vi "Handle EStop.vi"(8 "error in (no error)":errorcluster, 10 "Temp. Input":dbl, 11 "Tag Name":string) -> (0 "error out":errorcluster, 2 "History Data":T1(array[cluster]))   [LabVIEW 2023]
uses:
  8fdf3798-820e-43b9-bbcf-a8150b0dfc24.vi
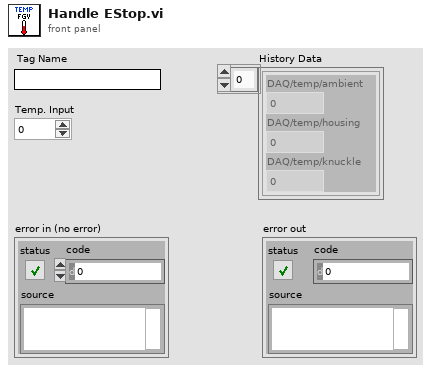
[diagram p1: front panel]
types:
  T1 = cluster{"DAQ/temp/ambient":dbl, "DAQ/temp/housing":dbl, "DAQ/temp/knuckle":dbl}[]
  T2 = cluster{"DAQ/temp/ambient":dbl, "DAQ/temp/housing":dbl, "DAQ/temp/knuckle":dbl}
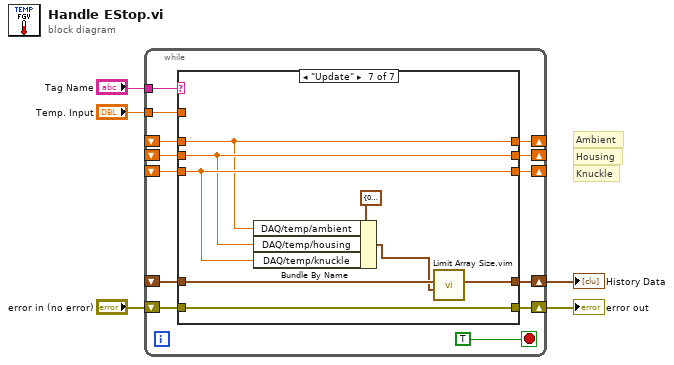
[diagram p0: block diagram]
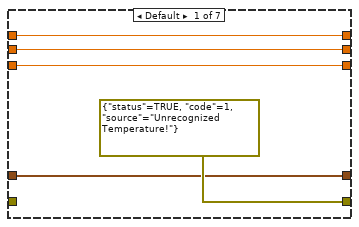
[diagram p2: hidden frame]
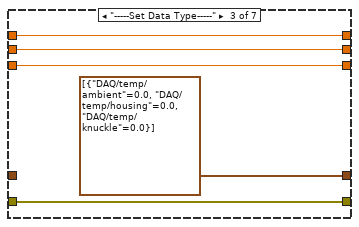
[diagram p4: hidden frame]
diagram:
  # "Knuckle"
  # "Housing"
  # "Ambient"
  n1 = while {
    tunnel: "Tag Name" -> [w14]
    shift-right: [w12] -> w2
    shift-left: _ -> [w13]
    shift-right: [w16] -> w4
    shift-left: "error in (no error)" -> [w17]
    shift-right: [w11] -> _
    shift-left: _ -> [w15]
    shift-right: [w10] -> _
    shift-left: _ -> [w7]
    shift-right: [w9] -> _
    shift-left: _ -> [w8]
    tunnel: "Temp. Input" -> [w6]
    stop <- TRUE stop-if-true
    n2 = case shown="\"Update\"" w14 {
      tunnel: w17 -> [_ w28 w33 w38 w43 w48 w56]
      tunnel: [errorcluster {"status"=TRUE, "code"=1, "source"="Unrecognized Temperature!"} ("error constant") w28 w33 w38 w43 w48 w56] -> w16
      tunnel: w15 -> [w21 w26 w31 _ w41 w47 w52]
      tunnel: w13 -> [w22 w27 _ w35 w40 w44 w51]
      tunnel: [w22 w27 T1 [{"DAQ/temp/ambient"=0.0, "DAQ/temp/housing"=0.0, "DAQ/temp/knuckle"=0.0}] ("History Data") w35 w40 w44 w49] -> w12
      tunnel: [w21 w26 w31 w34 w41 w47 w52] -> w11
      tunnel: [w19 w24 w29 w36 w42 w45 w54] -> w10
      tunnel: [w20 w25 w30 w37 w39 w46 w53] -> w9
      tunnel: w8 -> [w20 w25 w30 w37 _ w46 w53]
      tunnel: w7 -> [w19 w24 w29 w36 w42 _ w54]
      tunnel: w6 -> [_ _ _ w34 w39 w45 _]
      frame Default {
      }
      frame "" {
      }
      frame "-----Set Data Type-----" {
      }
      frame "DAQ/temp/ambient" {
      }
      frame "DAQ/temp/housing" {
      }
      frame "Temp/actual" {
      }
      frame "Update" {
        n3 = Bundle By Name(cluster=T2 {"DAQ/temp/ambient"=0.0, "DAQ/temp/housing"=0.0, "DAQ/temp/knuckle"=0.0}, "DAQ/temp/ambient"=w52, "DAQ/temp/housing"=w53, "DAQ/temp/knuckle"=w54) -> (w50:T2)
        n4 = call "Limit Array Size.vim"("Numeric"=w50, "Array in"=w51) -> ("Array out"=w49:T1)  [unwired: 5 in]
      }
    }
  }
  "error out" <- w4
  "History Data" <- w2
